vi "Info.vi"(8 "error in (no error)":errorcluster, 11 "MDPtrMgr in":refnum<class "MDPtrMgr.lvclass">) -> (0 "error out":errorcluster, 1 "# free MDPtrs in caches":i32, 2 "# MDPtrs allocated":i32, 3 "MDPtrMgr out":refnum<class "MDPtrMgr.lvclass">, 4 "# caches":i32)   [LabVIEW 2017, in "MDPtr.lvlib" / "MDPtrMgr.lvclass"]
uses:
  MDPtrMgr.lvclass
  MDPtrMgr.lvclass/MDPtrMgr.ctl
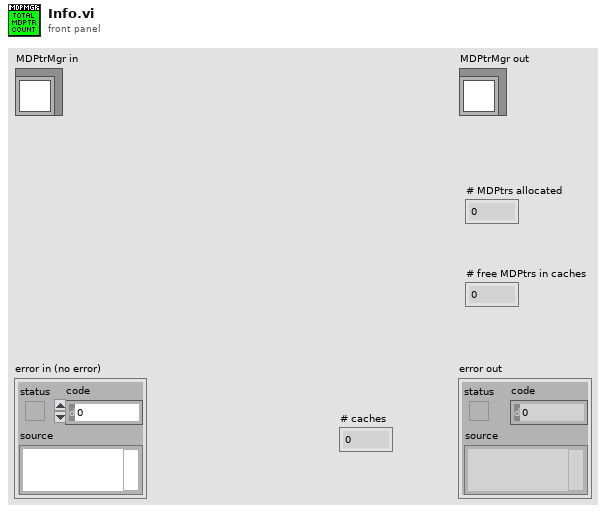
[diagram p1: front panel]
types:
  T1 = typedef "MDPtr.lvlib/MDPtrMgr.lvclass/Def-MDPtrQ.ctl" = refnum<queue>
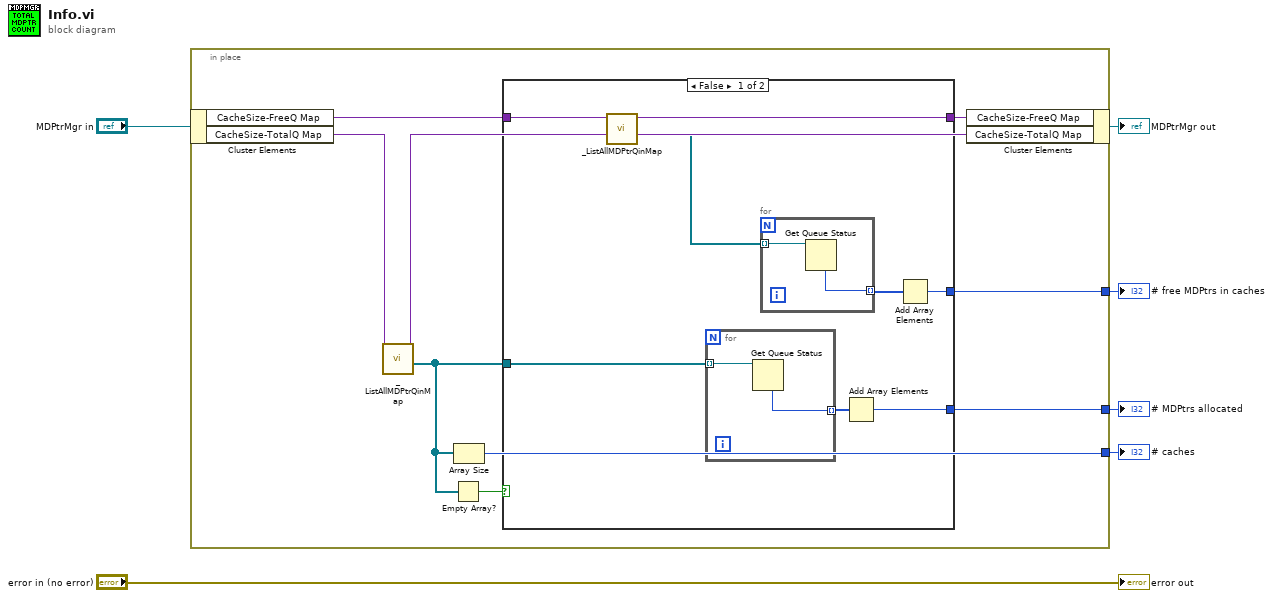
[diagram p0: block diagram]
diagram:
  n1 = in-place "In Place Element Structure" {
    in-place-border: [w13] -> w3
    in-place-border: [w12] -> w2
    in-place-border: [w7] -> w1
    n2 = in-place-cluster #1("MDPtrMgr in") -> ("CacheSize-FreeQ Map"=w8:variant, "CacheSize-TotalQ Map"=w15:variant)
    n3 = call "_ListAllMDPtrQinMap.vi"("Variant in"=w15) -> ("Array"=w10:T1[], "Variant"=w14:variant)  [unwired: 8 in, 1 out]
    n4 = Empty Array?(array=w10) -> (empty?=w11:bool)
    n5 = Array Size(array=w10) -> (size(s)=w12:i32)
    n6 = case shown="False" w11 {
      tunnel: [w22 _] -> w13
      tunnel: w10 -> [w21 _]
      tunnel: [w18 w28] -> w9
      tunnel: w8 -> [w19 w28]
      tunnel: [w17 _] -> w7
      frame False {
        n7 = call "_ListAllMDPtrQinMap.vi"("Variant in"=w19) -> ("Array"=w16:T1[], "Variant"=w18:variant)  [unwired: 8 in, 1 out]
        n8 = for {
          tunnel: w21 -> [w27] mode=indexing
          tunnel: [w26] -> w23 mode=indexing
          n9 = Get Queue Status(queue=w27) -> (# elements in queue=w26:i32)  [unwired: 2 in, 7 out]
        }
        n10 = for {
          tunnel: w16 -> [w25] mode=indexing
          tunnel: [w24] -> w20 mode=indexing
          n11 = Get Queue Status(queue=w25) -> (# elements in queue=w24:i32)  [unwired: 2 in, 7 out]
        }
        n12 = Add Array Elements(numeric array=w23) -> (sum=w22:i32)
        n13 = Add Array Elements(numeric array=w20) -> (sum=w17:i32)
      }
      frame True {
      }
    }
    n14 = in-place-cluster #1("CacheSize-FreeQ Map"=w9, "CacheSize-TotalQ Map"=w14) -> (→"MDPtrMgr out":refnum<class "MDPtrMgr.lvclass">)
  }
  "# MDPtrs allocated" <- w3
  "# caches" <- w2
  "# free MDPtrs in caches" <- w1
  "error out" <- "error in (no error)"
